vi "FGV Erweiterte Konfig.vi"(6 "Aktion":T10, 7 "Parameter Sensoren":T1 {"Druck Kalter Block" format="%#_5g"; "Offset Druck FTIR IAG" format="%#_5g"; "Offset Druck CG" format="%#_5g"; "Offset Druck CG PMA" format="%#_5g"; "Offset Durchfl.PMA" format="%#_5g"; "Offset Druck Umgebung" format="%#_5g"; "Offset Druck Ausgang" format="%#_5g"; "Offset Durchfl.FTIR" format="%#_5g"; "Kal.Durchfl.PMA" format="%.3g"; "Kal.Durchfl.FTIR" format="%.3g"}, 8 "Dichtheitstest?":bool, 9 "Sonstige":T3 {"ext. Befüllung" items=["Deaktiviert", "Aktiviert"]; "Dichtheitstest Umfang" items=["Pumpe / Filter / FT-IR / PNS", "Pumpe / Filter / FT-IR", "Filter / FT-IR", "FT-IR"]; "Befüllung aktiv" items=["Deaktiviert", "Aktiviert"]}, 10 "Aktionen Dichtheitstest":T2, 11 "PID-Parameter Anzeige":T7 {"Heizung\nHeizleitungen"."max. OUT" format="%#_5g"; "Heizung\nHeizleitungen"."Regelzonengr." format="%#_5g"; "Heizung\nHeizleitungen"."D-Anteil" format="%#_5g"; "Heizung\nHeizleitungen"."I-Anteil" format="%#_5g"; "Heizung\nHeizleitungen"."P-Anteil" format="%.1f"; "Heizleitung\nExtern"."max. OUT" format="%#_5g"; "Heizleitung\nExtern"."Regelzonengr." format="%#_5g"; "Heizleitung\nExtern"."D-Anteil" format="%#_5g"; "Heizleitung\nExtern"."I-Anteil" format="%#_5g"; "Heizleitung\nExtern"."P-Anteil" format="%.1f"; "Heizung\nFB-Druckregler"."max. OUT" format="%#_5g"; "Heizung\nFB-Druckregler"."Regelzonengr." format="%#_5g"; "Heizung\nFB-Druckregler"."D-Anteil" format="%#_5g"; "Heizung\nFB-Druckregler"."I-Anteil" format="%#_5g"; "Heizung\nFB-Druckregler"."P-Anteil" format="%.1f"; "Heizung\nPumpe"."max. OUT" format="%#_5g"; "Heizung\nPumpe"."Regelzonengr." format="%#_5g"; "Heizung\nPumpe"."D-Anteil" format="%#_5g"; "Heizung\nPumpe"."I-Anteil" format="%#_5g"; "Heizung\nPumpe"."P-Anteil" format="%.1f"; "Heizung\nFilterblock"."max. OUT" format="%#_5g"; "Heizung\nFilterblock"."Regelzonengr." format="%#_5g"; "Heizung\nFilterblock"."D-Anteil" format="%#_5g"; "Heizung\nFilterblock"."I-Anteil" format="%#_5g"; "Heizung\nFilterblock"."P-Anteil" format="%.1f"}) -> (0 "Dichtheitstest?":bool, 1 "Sonstige":T3 {"ext. Befüllung" items=["Deaktiviert", "Aktiviert"]; "Dichtheitstest Umfang" items=["Pumpe / Filter / FT-IR / PNS", "Pumpe / Filter / FT-IR", "Filter / FT-IR", "FT-IR"]; "Befüllung aktiv" items=["Deaktiviert", "Aktiviert"]}, 2 "Aktionen Dichtheitstest":T2, 3 "PID-Parameter Anzeige":T7 {"Heizung\nHeizleitungen"."max. OUT" format="%#_5g"; "Heizung\nHeizleitungen"."Regelzonengr." format="%#_5g"; "Heizung\nHeizleitungen"."D-Anteil" format="%#_5g"; "Heizung\nHeizleitungen"."I-Anteil" format="%#_5g"; "Heizung\nHeizleitungen"."P-Anteil" format="%.1f"; "Heizleitung\nExtern"."max. OUT" format="%#_5g"; "Heizleitung\nExtern"."Regelzonengr." format="%#_5g"; "Heizleitung\nExtern"."D-Anteil" format="%#_5g"; "Heizleitung\nExtern"."I-Anteil" format="%#_5g"; "Heizleitung\nExtern"."P-Anteil" format="%.1f"; "Heizung\nFB-Druckregler"."max. OUT" format="%#_5g"; "Heizung\nFB-Druckregler"."Regelzonengr." format="%#_5g"; "Heizung\nFB-Druckregler"."D-Anteil" format="%#_5g"; "Heizung\nFB-Druckregler"."I-Anteil" format="%#_5g"; "Heizung\nFB-Druckregler"."P-Anteil" format="%.1f"; "Heizung\nPumpe"."max. OUT" format="%#_5g"; "Heizung\nPumpe"."Regelzonengr." format="%#_5g"; "Heizung\nPumpe"."D-Anteil" format="%#_5g"; "Heizung\nPumpe"."I-Anteil" format="%#_5g"; "Heizung\nPumpe"."P-Anteil" format="%.1f"; "Heizung\nFilterblock"."max. OUT" format="%#_5g"; "Heizung\nFilterblock"."Regelzonengr." format="%#_5g"; "Heizung\nFilterblock"."D-Anteil" format="%#_5g"; "Heizung\nFilterblock"."I-Anteil" format="%#_5g"; "Heizung\nFilterblock"."P-Anteil" format="%.1f"}, 5 "Parameter Sensoren":T1 {"Druck Kalter Block" format="%#_5g"; "Offset Druck FTIR IAG" format="%#_5g"; "Offset Druck CG" format="%#_5g"; "Offset Druck CG PMA" format="%#_5g"; "Offset Durchfl.PMA" format="%#_5g"; "Offset Druck Umgebung" format="%#_5g"; "Offset Druck Ausgang" format="%#_5g"; "Offset Durchfl.FTIR" format="%#_5g"; "Kal.Durchfl.PMA" format="%.3g"; "Kal.Durchfl.FTIR" format="%.3g"})   [LabVIEW 2020, in "Erweiterte Konfig.lvlib"]
uses:
  Erweiterte Konfig.lvlib
  FGV PID Aktionen.ctl
  PID-Parameter Anzeige.ctl
  PID-Parameter.ctl
  Visualisierungs Elemente/Zahlen-Eingabefeld.ctl
  Sonstige Parameter.ctl
  Visualisierungs Elemente/Auswahlfeld.ctl
  Log Konfig/Auswahlfeld aktiviert-deaktiviert.ctl
  Dichtheitstest Umfang.ctl
  Aktionen Dichtheitstest.ctl
  Parameter Sensoren.ctl
  Log Konfig/LogKonfig.lvlib
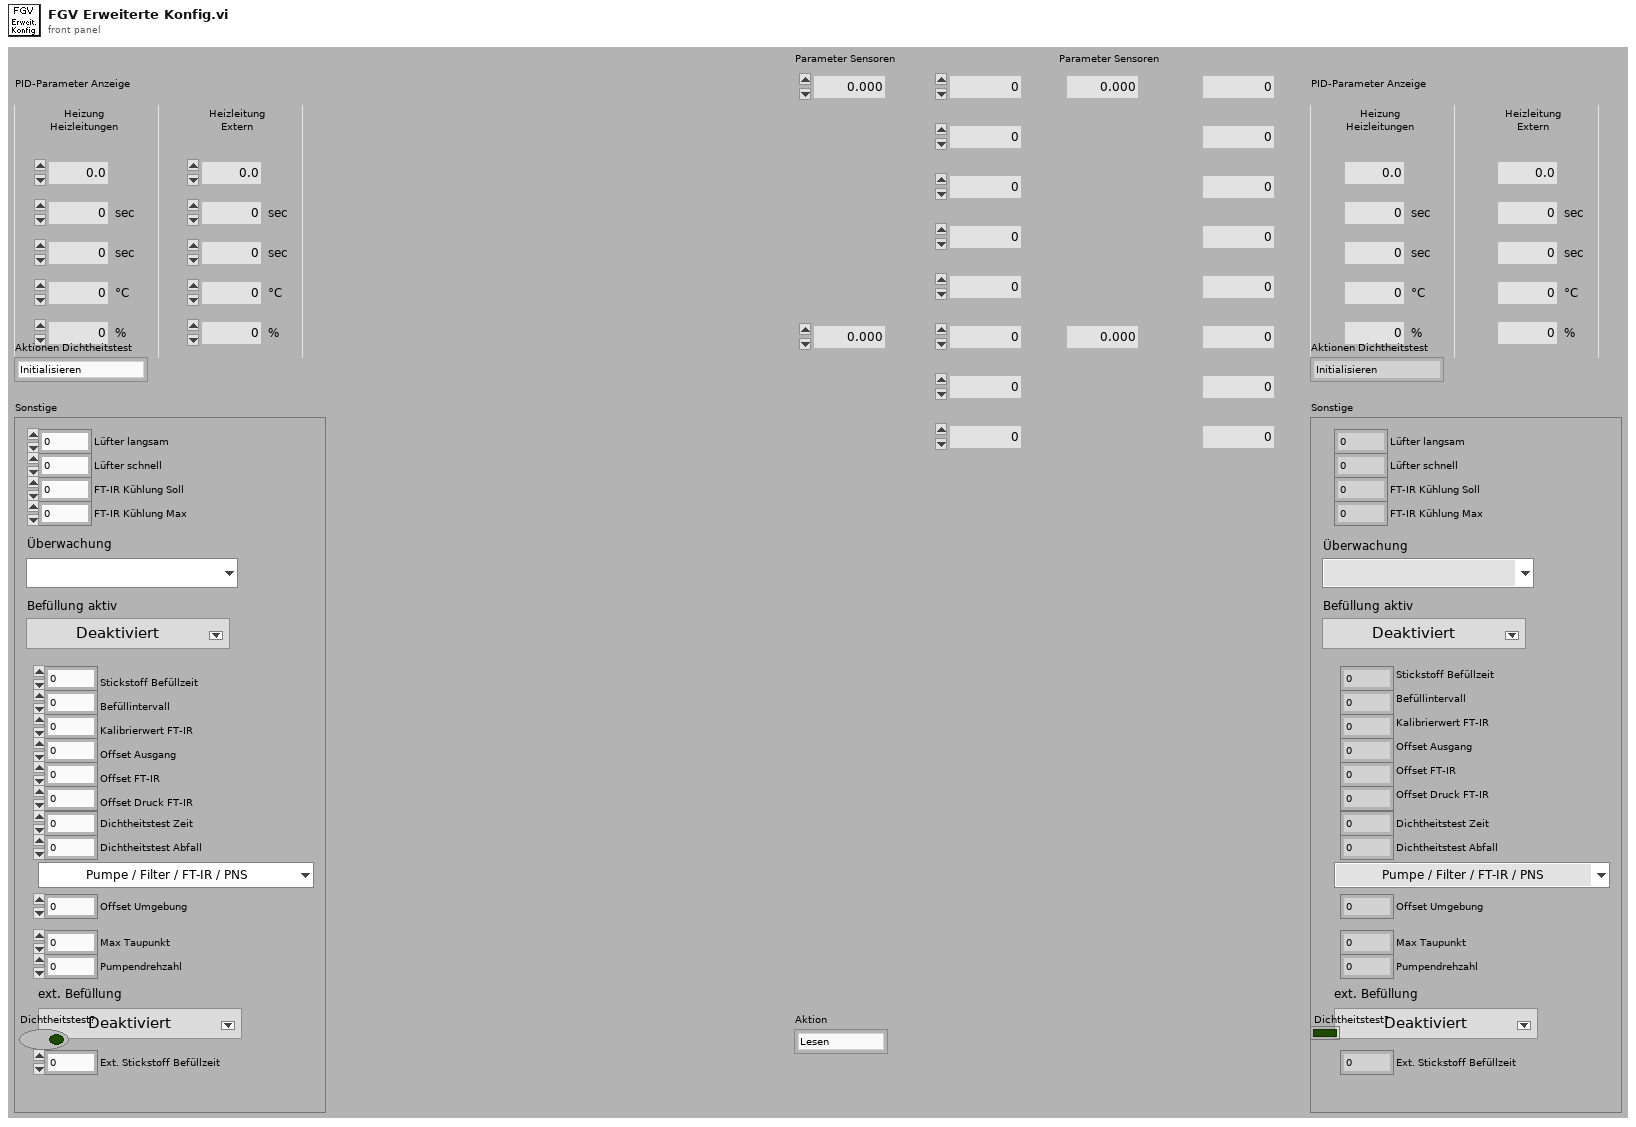
[diagram p1: front panel]
types:
  T1 = typedef "Erweiterte Konfig.lvlib/Parameter Sensoren.ctl" = cluster{"Kal.Durchfl.FTIR":sgl, "Kal.Durchfl.PMA":sgl, "Offset Durchfl.FTIR":sgl, "Offset Druck Ausgang":sgl, "Offset Druck Umgebung":sgl, "Offset Durchfl.PMA":sgl, "Offset Druck CG PMA":sgl, "Offset Druck CG":sgl, "Offset Druck FTIR IAG":sgl, "Druck Kalter Block":sgl}
  T2 = typedef "Erweiterte Konfig.lvlib/Aktionen Dichtheitstest.ctl" = enum16{"Initialisieren", "Unterdruck aufbauen", "Prop schließen", "Warten", "Auswertung", "Fertig"}
  T3 = typedef "Erweiterte Konfig.lvlib/Sonstige Parameter.ctl" = cluster{"Lüfter langsam":sgl, "Lüfter schnell":sgl, "FT-IR Kühlung Soll":sgl, "FT-IR Kühlung Max":sgl, "Überwachung":T4, "Befüllung aktiv":T5, "Stickstoff Befüllzeit":sgl, "Befüllintervall":sgl, "Kalibrierwert FT-IR":sgl, "Offset Ausgang":sgl, "Offset FT-IR":sgl, "Offset Druck FT-IR":sgl, "Dichtheitstest Zeit":sgl, "Dichtheitstest Abfall":sgl, "Dichtheitstest Umfang":T6, "Offset Umgebung":sgl, "Max Taupunkt":sgl, "Pumpendrehzahl":sgl, "ext. Befüllung":T5, "Ext. Stickstoff Befüllzeit":sgl}
  T4 = typedef "Auswahlfeld.ctl" = u16
  T5 = typedef "LogKonfig.lvlib/Auswahlfeld aktiviert-deaktiviert.ctl" = u16
  T6 = typedef "Erweiterte Konfig.lvlib/Dichtheitstest Umfang.ctl" = u16
  T7 = typedef "Erweiterte Konfig.lvlib/PID-Parameter Anzeige.ctl" = cluster{"Heizung\nFilterblock":T8, "Heizung\nPumpe":T8, "Heizung\nHeizleitungen":T8, "Heizleitung\nExtern":T8, "Heizung\nFB-Druckregler":T8}
  T8 = typedef "Erweiterte Konfig.lvlib/PID-Parameter.ctl" = cluster{"P-Anteil":T9, "I-Anteil":T9, "D-Anteil":T9, "Regelzonengr.":T9, "max. OUT":T9}
  T9 = typedef "Zahlen-Eingabefeld.ctl" = sgl
  T10 = typedef "Erweiterte Konfig.lvlib/FGV PID Aktionen.ctl" = enum16{"Lesen", "Schreiben PID", "Schreiben Sonstige", "Dichtheitstest", "Aktionen Dicht.", "Parameter Sensor"}
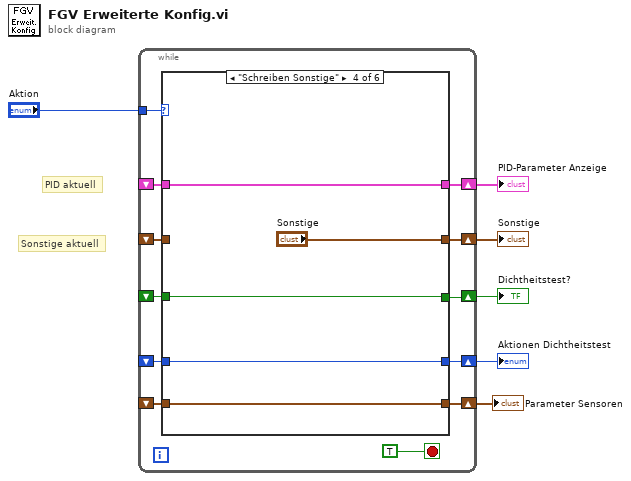
[diagram p0: block diagram]
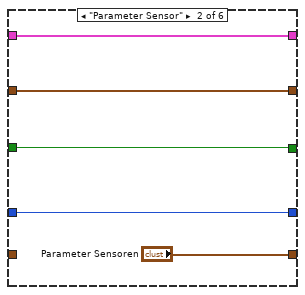
[diagram p3: hidden frame]
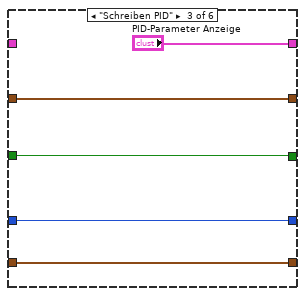
[diagram p4: hidden frame]
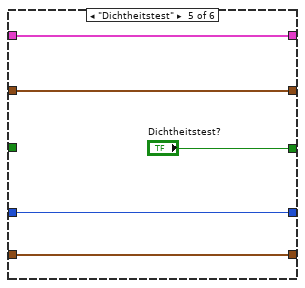
[diagram p5: hidden frame]
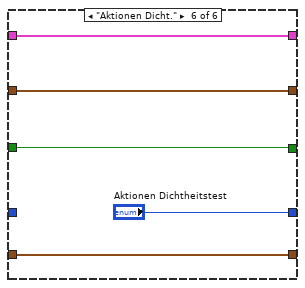
[diagram p6: hidden frame]
diagram:
  # "Sonstige aktuell"
  # "PID aktuell"
  n1 = while {
    tunnel: "Aktion" -> [w17]
    shift-right: [w16] -> w5
    shift-left: _ -> [w15]
    shift-right: [w14] -> w4
    shift-left: _ -> [w13]
    shift-right: [w12] -> w3
    shift-left: _ -> [w11]
    shift-right: [w10] -> w2
    shift-left: _ -> [w9]
    shift-right: [w8] -> w1
    shift-left: _ -> [w7]
    stop <- TRUE stop-if-true
    n2 = case shown="\"Schreiben Sonstige\"" w17 {
      tunnel: [w23 w28 "PID-Parameter Anzeige" w38 w41 w45] -> w16
      tunnel: w15 -> [w23 w28 _ w38 w41 w45]
      tunnel: [w22 w27 w32 "Sonstige" w42 w46] -> w14
      tunnel: w13 -> [w22 w27 w32 _ w42 w46]
      tunnel: [w21 w26 w31 w36 "Dichtheitstest?" w47] -> w12
      tunnel: w11 -> [w21 w26 w31 w36 _ w47]
      tunnel: [w20 w25 w30 w35 w40 "Aktionen Dichtheitstest"] -> w10
      tunnel: w9 -> [w20 w25 w30 w35 w40 _]
      tunnel: [w19 "Parameter Sensoren" w29 w34 w39 w44] -> w8
      tunnel: w7 -> [w19 _ w29 w34 w39 w44]
      frame "Lesen", Default {
      }
      frame "Parameter Sensor" {
      }
      frame "Schreiben PID" {
      }
      frame "Schreiben Sonstige" {
      }
      frame "Dichtheitstest" {
      }
      frame "Aktionen Dicht." {
      }
    }
  }
  "PID-Parameter Anzeige" <- w5
  "Sonstige" <- w4
  "Dichtheitstest?" <- w3
  "Aktionen Dichtheitstest" <- w2
  "Parameter Sensoren" <- w1
